vi "Digilens DLP Gen2 UI .vi"(11 "TopLevel In":refnum<class "TopLevel.lvclass">) -> (3 "TopLevel Out":refnum<class "TopLevel.lvclass">)   [LabVIEW 2022 SP3, in "TopLevel.lvclass"] (continued)
  T26 = typedef "TopLevel.lvclass/API Command Enum.ctl" = enum16{"Execute Printer Commands", "Pre Purge", "Enable Ink Ch-1", "Enable Ink Ch-2", "Enable Ink Ch-3", "Enable Ink Ch-4", "Enable Ink Ch-5", "Enable Ink Ch-6", "Disable Ink Ch-1", "Disable Ink Ch-2", "Disable Ink Ch-3", "Disable Ink Ch-4", "Disable Ink Ch-5", "Disable Ink Ch-6", "ExecuteIdlePrintCycle", "StopIdlePrintCycle", "Abort", "LoadDLP2GUIConfig", "SaveDLP2GUIConfig", "PrimingMode", "SetHeadTemperature", "EnableHead", "EnableHeadHeat", "SetSystemMode", "HeadPrint", "AbortAll", "Send Printer String", "WriteInitXML"}
  T27 = typedef "TopLevel.lvclass/PrimingMode APIData.ctl" = cluster{"Interval (s)":dbl, "PurgeDuration (s)":dbl, "Repeats":u8, "PrimingMode":T13, "Head":T18, "Frequency (Hz)":i32, "PrintWeight":dbl}
  T28 = typedef "PrintCmdParameters--Cluster.ctl" = cluster{"Command File Path":path, "No. of Print Repeats":i32, "HomeOnComplete":bool}
  T29 = typedef "TopLevel.lvclass/API Command Cluster.ctl" = cluster{"Command":T26, "Arguments":string, "Data":variant}
  T30 = typedef "IdlePrintCmdParameters--Cluster.ctl" = cluster{"Command File Path":path, "IdleMode":bool, "IdleCycleInterval(s)":dbl}
  T31 = typedef "IO.lvclass/ICP2-DO Channel Names.ctl" = enum16{"None", "Meniscus Valve Open - R1", "Meniscus Valve Open - R2", "Meniscus Valve Open - R3", "Meniscus Valve Open - R4", "Meniscus Valve Open - R5", "Meniscus Valve Open - R6", "Ink Flow Valve Open - R1", "Ink Flow Valve Open - R2", "Ink Flow Valve Open - R3", "Ink Flow Valve Open - R4", "Ink Flow Valve Open - R5", "Ink Flow Valve Open - R6", "SW_LED - Ink Valve - R1", "SW_LED - Ink Valve - R2", "SW_LED - Ink Valve - R3", "Recirc Pump On - R1", "Recirc Pump On - R2", "Recirc Pump On - R3", "Recirc Pump On - R4", "Recirc Pump On - R5", "Recirc Pump On - R6", "SW_LED - Ink Valve - R4", "SW_LED - Ink Valve - R5", "SW_LED - Ink Valve - R6"}
  T32 = enum32{"invalid app kind", "Development System", "Run Time System", "Student Edition", "Embedded LabVIEW", "Evaluation", "Custom"}
  T33 = typedef "printWeights--cluster.ctl" = cluster{"Weights 1":dbl, "Weights 2":dbl, "Weights 3":dbl, "Weights 4":dbl, "Weights 5":dbl, "Weights 6":dbl}
  T34 = typedef "Imageresolution--cluster.ctl" = cluster{"X Resolution":i32, "Y Resolution":i32}
  T35 = typedef "TD MasterConfiguration DLPC2--cluster.ctl" = cluster{"Paths":T36, "ColorPaneMapping":T37, "Materials":string[], "ColorPlanes":string[], "SpitVoltages_Half":T39, "SpitVoltages_Full":T39, "SystemMode":string[], "PrimeModeConfig":T27[], "Running Average Duration_s":dbl}
  T36 = typedef "DLPC2_Path--Cluster.ctl" = cluster{"DigiBit WG Design Folder":path, "Compensated GS Image Folder":path, "Nozzle GS Files Head 1":path, "Nozzle GS Files Head 2":path, "Nozzle GS Files Head 3":path, "Nozzle GS Files Head 4":path, "Nozzle GS Files Head 5":path, "Nozzle GS Files Head 6":path}
  T37 = typedef "TD HeadColorPaneMappingAll--cluster.ctl" = cluster{"Head 1":T38, "Head 2":T38, "Head 3":T38, "Head 4":T38, "Head 5":T38, "Head 6":T38}
  T38 = typedef "TD HeadColorPaneMapping--cluster.ctl" = cluster{"Material":string, "ColorPane":string}
  T39 = typedef "SpitVoltages--Cluster.ctl" = cluster{"1":dbl, "2":dbl, "3":dbl, "4":dbl, "5":dbl, "6":dbl}
  T40 = typedef "Motor Controller.lvclass/Status.ctl" = cluster{"Motor Controller Config Data":T41, "Motor Controller Data":cluster{"Enabled?":bool}, "Stage Move":T42, "Stage Busy?":bool}
  T41 = typedef "Motor Controller.lvclass/Motor Controller Config Data.ctl" = cluster{"Motor IP Addresss":string, "Current Position":i32, "Pulse_Per_mm":i32, "PrePrint":dbl[], "Load Position_mm":i32, "Laminate Position_mm":i32}
  T42 = typedef "Motor Controller.lvclass/Stage Move Data.ctl" = cluster{"Current Step":string, "Move Data":T43[]}
  T43 = typedef "Motor Controller.lvclass/Batch Index Speed Data.ctl" = cluster{"Batch & Cycle":string, "Move":cluster{"Index_mm":i32, "Speed_mm_s":i32}, "Status":T44}
  T44 = typedef "Motor Controller.lvclass/Move Status.ctl" = enum16{"Pending", "In Progress", "Completed"}
  T45 = enum8{"Enabled", "Disabled", "Disabled and Grayed Out"}
  T46 = enum32{"Invalid", "Standard", "Closed", "Hidden", "Minimized", "Maximized"}
  T47 = typedef "LoadImagesData--cluster.ctl" = cluster{"Images[]":path[], "Calibration":bool}
  T48 = typedef "PythonVersion--Enum.ctl" = enum16{"3.9 64", "3.9 32", "3.12 64", "3.12 32"}
  T49 = typedef "SeperateLayersPython--cluster.ctl" = cluster{"Path_to_Tiff":path, "OutputFolder":path, "DPI_x":i32, "DPI_y":i32, "Python_Version":T48}
  T50 = typedef "IO.lvclass/ICP1-AO Channel Names.ctl" = enum16{"None", "Meniscus Pressure Set - R1", "Meniscus Pressure Set - R2", "Meniscus Pressure Set - R3", "Meniscus Pressure Set - R4", "Meniscus Pressure Set - R5", "Meniscus Pressure Set - R6", "Meniscus Vac Pump Speed"}
  T51 = typedef "TopLevel.lvclass/Digilens Config Cluster.ctl" = cluster{"Motion Controller":T41, "IO Config":T52, "PrinterConfiguration":T55, "DAQ Settings":T56}
  T52 = typedef "IO.lvclass/IO Config Data.ctl" = cluster{"DAQDevices":T53[], "DI Channels":T54[], "DO Channels":T54[], "Material Names":string[], "AI Channels":T54[], "AO Channels":T54[]}
  T53 = typedef "IO.lvclass/DCON_DeviceConfig--Cluster.ctl" = cluster{"COM":string, "DeviceName":string, "BaudRate":u32, "Number of Channels":i32, "DeviceAddress":i32, "Enable":bool}
  T54 = typedef "IO.lvclass/Channel Data.ctl" = cluster{"Channel Name":string, "Device Name":string, "Channel No":string}
  T55 = typedef "GIS Printer.lvclass/PrinterConfiguration--Cluster.ctl" = cluster{"IPAddress":string, "Move Stage on RTP Command?":bool, "Stage Move Position":string, "PH1-Prime Path":path, "PH2-Prime Path":path, "PH3-Prime Path":path, "PH4-Prime Path":path, "PH5-Prime Path":path, "PH6-Prime Path":path, "PrintScriptsFolder":path, "PurgeScriptsFolder":path, "StageScriptsFolder":path, "PH1-HeatOn Path":path, "PH2-HeatOn Path":path, "PH3-HeatOn Path":path, "PH4-HeatOn Path":path, "PH5-HeatOn Path":path, "PH6-HeatOn Path":path, "PH1-HeatOff Path":path, "PH2-HeatOff Path":path, "PH3-HeatOff Path":path, "PH4-HeatOff Path":path, "PH5-HeatOff Path":path, "PH6-HeatOff Path":path}
  T56 = typedef "DAQ.lvclass/TD DAQ Settings--cluster.ctl" = cluster{"Simulate DAQ":bool, "DI Settings":T57[], "AI Settings":T58[], "Relay IONames":string[], "AO IONames":string[], "AO NChan SingleTask":bool}
  T57 = typedef "DAQ.lvclass/TD DI Instrument Settings--cluster.ctl" = cluster{"Disable":bool, "DI TaskName":string, "DI RefreshIntv":i32}
  T58 = typedef "DAQ.lvclass/TD AI Instrument Settings--cluster.ctl" = cluster{"Disable":bool, "AI TaskName":string, "AI InstSettings":T59, "SimAI Ranges":T60}
  T59 = typedef "DAQ.lvclass/TD AI InstSettings--cluster.ctl" = cluster{"DaqRate":dbl, "NumSamples":i32}
  T60 = typedef "DAQ.lvclass/TD SimAI Ranges--cluster.ctl" = cluster{"lo":dbl, "hi":dbl}
  T61 = typedef "DLPConfig_Initialization.ctl" = cluster{"PrinterInitialization":cluster{"Printer":cluster{"#attributes":cluster{"Name":string}}, "VacPumpSet":cluster{"#attributes":cluster{"VacPumpEnable":bool, "VacPumpSpeed":dbl}}, "HIBEnable":cluster{"#attributes":cluster{"HIB1Enable":bool, "HIB2Enable":bool, "HIB3Enable":bool, "HIB4Enable":bool, "HIB5Enable":bool, "HIB6Enable":bool}}, "PrinterCompensation":T62}, "HeadSet":cluster{"HeadProperties":T63[]}, "InkSet":cluster{"Ink":T65[]}, "Troubleshooting":cluster{"PMBLogging":cluster{"#attributes":cluster{"PMBMonitorDuringPrint":bool, "PMBMonitorDuringIdle":bool, "LogSwatheInputData":bool, "LogSwatheOutputData":bool, "LogPrintheadColourPlanes":bool, "LogPMBCommunication":bool, "LogSimulatedOutput":bool, "LogAllPMBCommunicationData":bool, "LogPMBSpace":bool, "ExtendedPMBSpaceLogging":bool, "LogPMBWriteSpeed":bool, "LogUsbRetries":bool}}, "HIBLogging":cluster{"#attributes":cluster{"HIBMonitoringDuringPrint":bool, "HIBMonitoringLog":bool}}}}
  T62 = typedef "DLP2_PrinterCompensationProperties.ctl" = cluster{"#attributes":cluster{"AppName":string, "PrintWeightMultiplier":dbl, "Rotation":bool, "Driver":string, "Server":string, "Database":string, "User":string, "Password":string}}
  T63 = typedef "DLP2_PrinterHeadProperties.ctl" = cluster{"#attributes":T64}
  T64 = typedef "DLPConfig)Init_HeadPropertyAttr--Cluster.ctl" = cluster{"HeadNumber":u8, "Material":string, "HeadLocalX":dbl, "HeadLocalY":dbl, "HeadRotationAngle":dbl, "VH2L_Hi":dbl, "VH2R_Hi":dbl, "VH1LA_Hi":dbl, "VH1LB_Hi":dbl, "VH1RA_Hi":dbl, "VH1RB_Hi":dbl, "VH2L_Lo":dbl, "VH2R_Lo":dbl, "VH1LA_Lo":dbl, "VH1LB_Lo":dbl, "VH1RA_Lo":dbl, "VH1RB_Lo":dbl}
  T65 = typedef "DLP2_PrinterMaterialProperties.ctl" = cluster{"#attributes":cluster{"InkType":string, "ColorPlane":string, "Heat":dbl, "Meniscus":dbl, "Recirculation":bool, "PrePrintPurge":bool, "PurgeTime":dbl, "PurgeCount":i32, "Density":dbl, "NumberofDrops":i32, "PrintWeight":dbl, "PrintheadPrime":bool}, "Idle":T66}
  T66 = typedef "InkIdleNodeConfigXML--Cluster.ctl" = cluster{"ShortIdle":cluster{"#attributes":cluster{"Heat":dbl, "Meniscus":dbl, "Recirculation":bool}}, "LongIdle":cluster{"#attributes":cluster{"Heat":dbl, "Meniscus":dbl, "Recirculation":bool}}}
  T67 = typedef "TopLevel.lvclass/Pre Purge Parameters.ctl" = cluster{"GIS File Path":path, "Duration (s)":dbl, "No. of Repeats":i32}
  T68 = typedef "RecipeInfo--Cluster.ctl" = cluster{"Path":path, "Type":string, "Product":string}
  T69 = typedef "TiffImageData--Cluster.ctl" = cluster{"ImageBufferMain":u8[][], "ChannelTargetMaterials":string[], "MaterialNames":string[]}
  T70 = typedef "GIS Status--Cluster.ctl" = cluster{"HeadEnabled":bool, "SpitEnabled":bool, "HeaterEnabled":bool, "TargetTemperature":dbl, "CurrentTemperature":dbl}
  T71 = typedef "HeadEnableStatus--cluster.ctl" = cluster{"PH1_Enable":bool, "PH2_Enable":bool, "PH3_Enable":bool, "PH4_Enable":bool, "PH5_Enable":bool, "PH6_Enable":bool}
  T72 = typedef "PersistentData--Cluster.ctl" = cluster{"ToolIdle":bool, "Meniscus Vac Pump Speed":dbl, "InkChEnable":cluster{"Enable Ink Ch-1":bool, "Enable Ink Ch-2":bool, "Enable Ink Ch-3":bool, "Enable Ink Ch-4":bool, "Enable Ink Ch-5":bool, "Enable Ink Ch-6":bool}, "HeatEnable":cluster{"Heater-1 Off":bool, "Heater-2 Off":bool, "Heater-3 Off":bool, "Heater-4 Off":bool, "Heater-5 Off":bool, "Heater-6 Off":bool}, "MiniscusPressure":cluster{"Meniscus Pressure Set - R1":dbl, "Meniscus Pressure Set - R2":dbl, "Meniscus Pressure Set - R3":dbl, "Meniscus Pressure Set - R4":dbl, "Meniscus Pressure Set - R5":dbl, "Meniscus Pressure Set - R6":dbl}, "RecircPumpFlow":cluster{"Recirc Pump Flow Set - R1":dbl, "Recirc Pump Flow Set - R2":dbl, "Recirc Pump Flow Set - R3":dbl, "Recirc Pump Flow Set - R4":dbl, "Recirc Pump Flow Set - R5":dbl, "Recirc Pump Flow Set - R6":dbl}}
  T73 = typedef "DLPConfig_RecipePrints.ctl" = cluster{"CellPrintRecipe":cluster{"#attributes":cluster{"Type":string, "RecipeName":string, "Product":string}, "CellPrint":cluster{"#attributes":cluster{"PrintImageFile":string, "PrintPass":i32, "PrintMode":string, "EncoderSource":string, "PrintGoSource":string, "DitheredSavePath":string, "GSSavePath":string}}[], "InkCompensationSet":cluster{"InkCompensation":cluster{"#attributes":cluster{"InkType":string, "Waveform":string, "ZoneCompensation":bool, "ZoneCompFile":string, "Overprint":dbl, "Bitmap":string, "SaveGSImg":bool, "GSSource":string, "GSValFile":string}}[]}}}
  T74 = typedef "DLPConfig_CalibrationPrints.ctl" = cluster{"CellPrintRecipe":cluster{"#attributes":cluster{"Type":string, "RecipeName":string, "Product":string}, "CellPrint":cluster{"#attributes":cluster{"PrintImageFile":string, "PrintPass":i32, "EncoderSource":string, "PrintGoSource":string, "Head":i32}}[], "InkCompensationSet":cluster{"InkCompensation":cluster{"#attributes":cluster{"InkType":string, "Waveform":string, "ZoneCompensation":bool}}[]}}}
  T75 = typedef "LoginEventData--CLuster.ctl" = cluster{"UserLevel":T76, "Login Time":timestamp}
  T76 = typedef "UserLevel--Enum.ctl" = enum16{"None", "Operator", "Engineer"}
  T77 = cluster{"Core":cluster{"Current VI Reference":refnum<vi>, "Close Panel on Exit?":bool}, "IO":refnum<class "IO.lvclass">, "GIS Printer":refnum<class "GIS Printer.lvclass">, "Motor Controller":refnum<class "Motor Controller.lvclass">, "Methods:Accessors:Digilens Config":T51, "Methods:Accessors:PrinterInitializationXML":T61, "Status":T40, "Exit Event":refnum<user-event>, "Purge\\PrePurge Channel Name":T19, "Pre Purge Parameters":T67, "API Command":T26, "TopLevel out":refnum<class "TopLevel.lvclass">, "Database":refnum<class "Database.lvclass">, "DLP2":refnum<class "DLP2.lvclass">, "DLP2Config":T35, "Materials":string[], "Color Panes":string[], "ConfigSaveRequired":bool, "DLP2ConfigLoaded":T35, "PrintDesign":T68, "DAQ":refnum<class "DAQ.lvclass">, "RGB Image":T6, "Planes Image":T6, "TIFFImageData":T69, "Image Resolution":T34, "Pre Purge API Data":T27, "Prime Names":cluster{"Prime 1":string, "Prime 2":string, "Prime 3":string, "Prime 4":string, "Prime 5":string, "Prime 6":string}, "Heater Enable":cluster{"HeaterEnblHead":T18, "Enable":bool}, "Head Temp ":cluster{"Head 1":cluster{"Actual":dbl, "Target":dbl}, "Head 2":cluster{"Actual":dbl, "Target":dbl}, "Head 3":cluster{"Actual":dbl, "Target":dbl}, "Head 4":cluster{"Actual":dbl, "Target":dbl}, "Head 5":cluster{"Actual":dbl, "Target":dbl}, "Head 6":cluster{"Actual":dbl, "Target":dbl}}, "GISHeadStatus":T70[], "SettingsUpdate":variant, "HeadStatus":T71, "Methods:Accessors:ConfigDict":T16, "Print":cluster{"RecipeXMLPath":path}, "SeparateLayers":T49, "PersistentData":T72, "HeadStatusPollData":T71, "CurrentDLPRecipe":T73, "CalibrationPrints":T74, "Login":T75, "PrintWeights":T33, "PrePrimeDone":bool, "PrePrimeTmrEnabled":bool, "PPP_Ditherered_Images":path[]}
  T78 = enum16{"Left Button", "Center Button", "Right Button", "Window Close"}
  T79 = typedef "eventvkey.ctl" = enum16{"ASCII", "Enter", "Return", "Shift", "Ctrl", "Alt", "Cmd", "Opt", "Caps", "NumLock", "Clear", "Break", "Up", "Down", "Left", "Right", "Insert", "Delete", "Home", "End", "PageUp", "PageDown", "Escape", "Help", "Pause", "ScrollLock", "F1", "F2", "F3", "F4", "F5", "F6", "F7", "F8", "F9", "F10", "F11", "F12", "F13", "F14", "F15", "F16", "F17", "F18", "F19", "F20", "F21", "F22", "F23", "F24", "Play", "VolumeUp", "VolumeDown", "Mute", "Two Byte Char"}
  T80 = typedef "NI_LVConfig.lvlib/Config Data RefNum.ctl" = refnum<k1>
  T81 = cluster{"#attributes":cluster{"PrintImageFile":string, "PrintPass":i32, "EncoderSource":string, "PrintGoSource":string, "Head":i32}}[]
  T82 = cluster{"PrintImageFile":string, "PrintPass":i32, "EncoderSource":string, "PrintGoSource":string, "Head":i32}
  T83 = typedef "TD Pathnames--cluster.ctl" = cluster{"RunTimeSys?":bool, "AppFolder":path, "ExecutablePath":path, "ConfigFolder":path, "DataLogFolder":path, "SystemLogFolder":path, "SeqFolder":path, "MainStartupPathname":path, "MainUIPathname":path, "SystemEventsFile":path, "SeqEventsFile":path, "Config SettingsFile":path, "DAQ IOConfigFile":path, "SystemSimulation":bool, "DLPUIConfigFile":path, "PrinterInitXMLFile":path, "PersistentXMLFile":path, "Error Log Folder":path, "RecipeXMLFolder":path, "CalibrationRecipeXMLFolder":path}
  T84 = typedef "DLP RecipeTypesData--Cluster.ctl" = cluster{"Product":string, "RecipePathsByProduct":path[], "RecipeNamesByProduct":string[]}
  T85 = typedef "DLP_MaterialToHeadMapping--Cluster.ctl" = cluster{"Head":u8, "Ink":T65}
  T86 = cluster{"Head 1":cluster{"Actual":dbl, "Target":dbl}, "Head 2":cluster{"Actual":dbl, "Target":dbl}, "Head 3":cluster{"Actual":dbl, "Target":dbl}, "Head 4":cluster{"Actual":dbl, "Target":dbl}, "Head 5":cluster{"Actual":dbl, "Target":dbl}, "Head 6":cluster{"Actual":dbl, "Target":dbl}}
  T87 = cluster{"Current VI Reference":refnum<vi>, "Close Panel on Exit?":bool}
  T88 = typedef "TopLevel.lvclass/UserEvents.ctl" = cluster{"API Incoming Event":refnum<user-event>, "API Executed Event":refnum<user-event>, "API Return Event":refnum<user-event>, "Exit Event":refnum<user-event>, "StatusChanged":refnum<user-event>, "DLP GUI Config Changed":refnum<user-event>, "AppEvent":refnum<user-event>, "Login Event":refnum<user-event>, "HeadPrimeStatusEvent":refnum<user-event>}
  T89 = cluster{"Prime 1":string, "Prime 2":string, "Prime 3":string, "Prime 4":string, "Prime 5":string, "Prime 6":string}
  T90 = typedef "Image Type" = u32
  T91 = enum8{"Enabled", "Disabled", "Disabled and Grayed Out"}[]
  T92 = cluster{"#attributes":cluster{"PrintImageFile":string, "PrintPass":i32, "PrintMode":string, "EncoderSource":string, "PrintGoSource":string, "DitheredSavePath":string, "GSSavePath":string}}[]
  T93 = cluster{"#attributes":cluster{"PrintImageFile":string, "PrintPass":i32, "PrintMode":string, "EncoderSource":string, "PrintGoSource":string, "DitheredSavePath":string, "GSSavePath":string}}
  T94 = typedef "DLP2.lvclass/Public Events--cluster.ctl" = cluster{"Temp01.AsyncCmd Event":refnum<user-event>, "Temp01.AsyncMsg Event":refnum<user-event>, "stop process":refnum<user-event>, "API Incoming Event":refnum<user-event>, "API Executed Event":refnum<user-event>, "API Return Event":refnum<user-event>, "Images":refnum<user-event>}
  T95 = typedef "Motor Controller.lvclass/UserEvents.ctl" = cluster{"API Incoming Event":refnum<user-event>, "API Executed Event":refnum<user-event>, "API Return Event":refnum<user-event>, "Status Changed Event":refnum<user-event>, "StopEvent":refnum<user-event>}
  T96 = typedef "IO.lvclass/UserEvents.ctl" = cluster{"API Incoming Event":refnum<user-event>, "API Executed Event":refnum<user-event>, "API Return Event":refnum<user-event>, "Status Changed Event":refnum<user-event>}
  T97 = typedef "GIS Printer.lvclass/UserEvents.ctl" = cluster{"API Incoming Event":refnum<user-event>, "API Executed Event":refnum<user-event>, "API Return Event":refnum<user-event>, "Status Changed Event":refnum<user-event>, "Abort":refnum<user-event>, "stop process":refnum<user-event>, "GISPollStatus":refnum<user-event>, "GISHeadStatus":refnum<user-event>, "Error Event":refnum<user-event>}
  T98 = cluster{"HIB1Enable":bool, "HIB2Enable":bool, "HIB3Enable":bool, "HIB4Enable":bool, "HIB5Enable":bool, "HIB6Enable":bool}
  T99 = typedef "processMode_parameters--cluster.ctl" = cluster{"Head Array":u8[], "ProcessHeat[]":dbl[], "ShortIdleHeat[]":dbl[], "LongIdleHeat[]":dbl[], "ProcessMeniscus[]":dbl[], "ShortIdleMeniscus[]":dbl[], "LongIdleMeniscus[]":dbl[], "ProcessRecirc[]":bool[], "ShortIdleRecirc[]":bool[], "LongIdleRecirc[]":bool[]}
  T100 = typedef "RecipesFolderSummary--Cluster.ctl" = cluster{"Products":string[], "RecipeTypes":string[]}
  T101 = typedef "TD IOCtrlUpdate.ctl" = cluster{"IOName":string, "vData":variant}
  T102 = typedef "DAQ.lvclass/TD PublicEvents--cluster.ctl" = cluster{"DaqOutputCmd Ev":refnum<user-event>, "stop process":refnum<user-event>, "DAQ.AsyncCmd Event":refnum<user-event>, "DAQStateChanged Event":refnum<user-event>, "DAQ.AsyncMsg Event":refnum<user-event>, "DAQ_DO_StatusEvent":refnum<user-event>, "DIStateChangeEv":refnum<user-event>, "UI StateChanged":refnum<user-event>, "PurgeTimerEvent":refnum<user-event>}
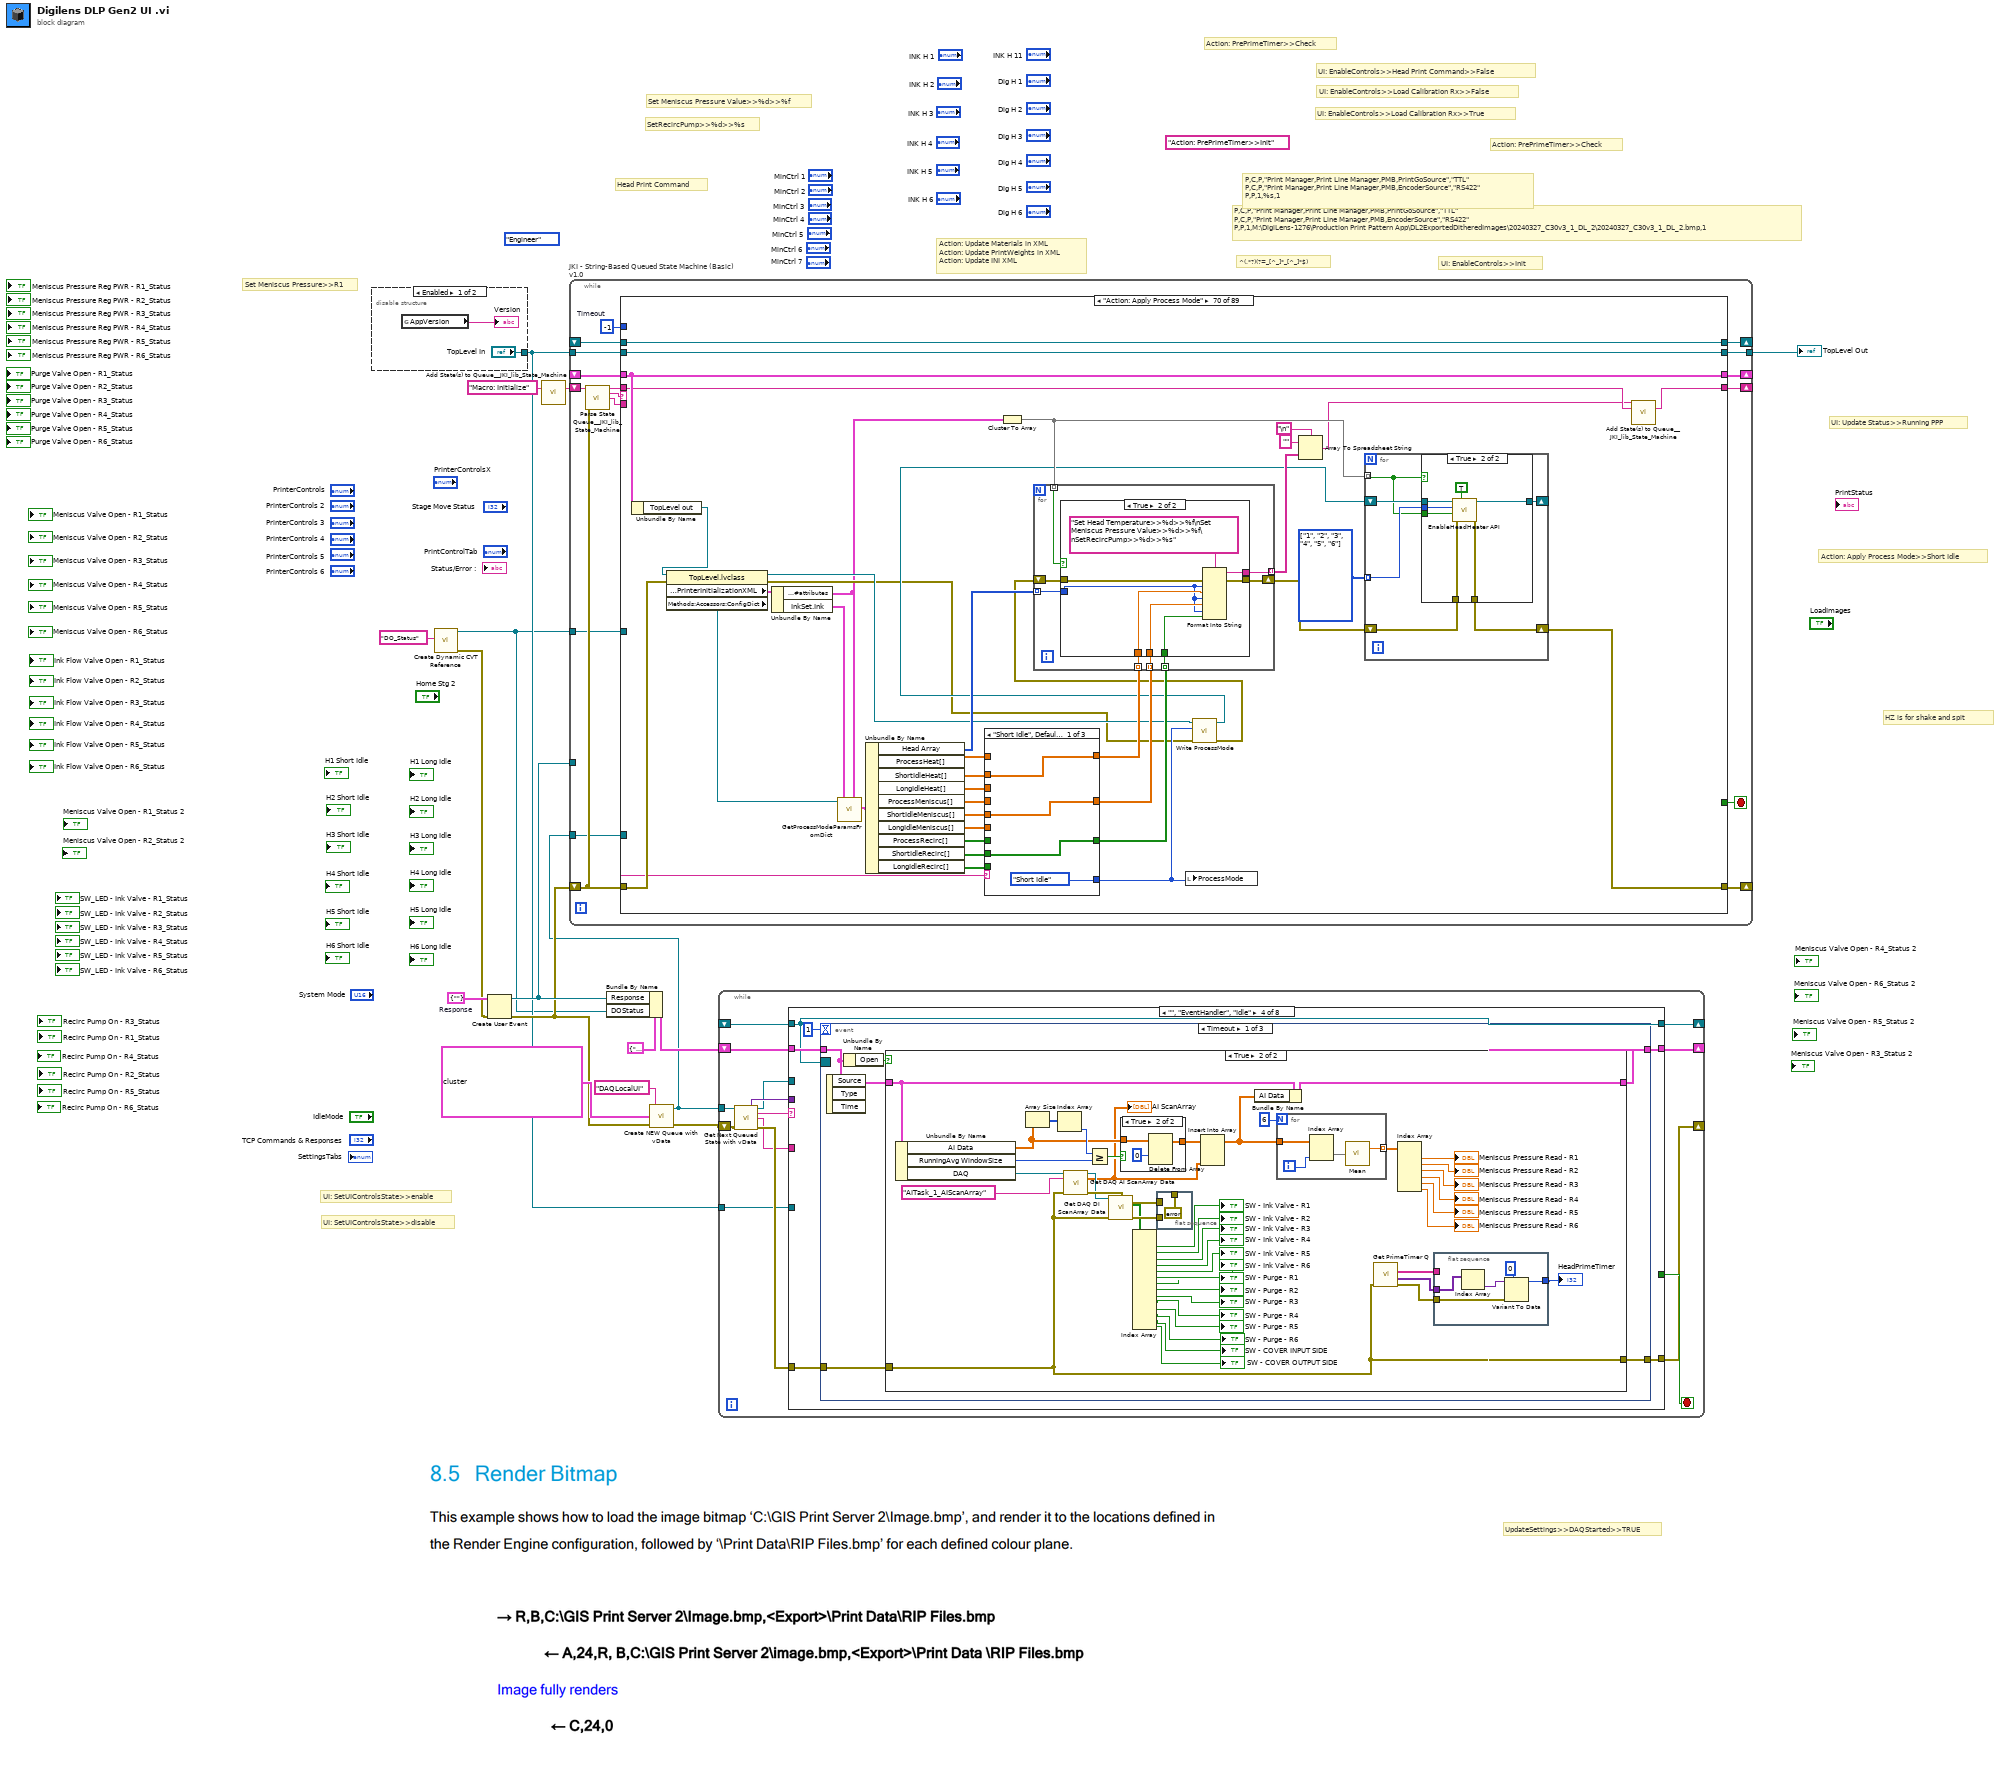
[diagram p0: block diagram]
diagram:
  (unwired) "Action: PrePrimeTimer>>Init" ("State(s) in Front (\"\")")
  (unwired) UserLevel_withoutNone--Enum."Engineer" ("UserLevel")
  w13 = cluster{"Response":string} {"Response"=""}  # Response
  # "SetRecircPump>>%d>>%s"
  # "Set Meniscus Pressure Value>>%d>>%f"
  # "Set Meniscus Pressure>>R1"
  # "Action: Apply Process Mode>>Short Idle"
  # "UI: Update Status>>Running PPP"
  # "UI: EnableControls>>Head Print Command>>False"
  # "Head Print Command"
  # "UI: EnableControls>>Load Calibration Rx>>False"
  # "Action: PrePrimeTimer>>Check"
  # "UI: EnableControls>>Init"
  # "Action: Update Materials in XML\nAction: Update PrintWeights in XML\nAction: Update INI XML"
  # "UI: EnableControls>>Load Calibration Rx>>True"
  # "Action: PrePrimeTimer>>Check"
  # "HZ is for shake and spit"
  # "P,C,P,\"Print Manager,Print Line Manager,PMB,PrintGoSource\",\"TTL\"\nP,C,P,\"Print Manager,Print Line Manager,PMB,EncoderSource\",\"RS422\"\nP,P,1,%s,1"
  # "P,C,P,\"Print Manager,Print Line Manager,PMB,PrintGoSource\",\"TTL\"\nP,C,P,\"Print Manager,Print Line Manager,PMB,EncoderSource\",\"RS422\"\nP,P,1,M:\\DigiLens-1276\\Production Print Pattern App\\DL2ExportedDitheredImages\\20240327_C30v3_1_DL_2\\20240327_C30v3_1_DL_2.bmp,1"
  # "^(.*?)(?=_[^_]*_[^_]*$)"
  # "UpdateSettings>>DAQStarted>>TRUE"
  # "UI: SetUIControlsState>>disable"
  # "UI: SetUIControlsState>>enable"
  n1 = disable-structure shown="Enabled" {
    disable-tunnel: ["TopLevel In" w19] -> w5
    frame Enabled {
      n2 = global read "GBL System.vi" "AppVersion"() -> (→"Version":string)
    }
    frame Disabled {
      n3 = call "Launcher.vi"() -> ("TopLevel out"=w19:refnum<class "TopLevel.lvclass">)  [unwired: 10 in, 1 out]
    }
  }
  n4 = call <vilib>:"Create Dynamic CVT Reference.vi"("DictName"="DO_Status") -> ("error out"=w3:errorcluster, "dCVT DVR out"=w2:T16)  [unwired: 9 in]
  n5 = Create User Event(user event datatype=w13, error in=w3) -> (user event=w7:refnum<user-event>, error out=w6:errorcluster)
  n6 = call <vilib>:"Add State(s) to Queue__JKI_lib_State_Machine.vi"("State(s) in (\"\")"="Macro: Initialize") -> ("States Out"=w16:string)  [unwired: 14 in]
  n7 = Bundle By Name(cluster=T17 {"String"="", "Response"=refnum, "Open"=FALSE, "DAQ"=refnum, "DOStatus"=refnum, "DIStateChangeEv"=refnum, "RunningAvg WindowSize"=0, "AI Data"=[]}, "Response"=w7, "DOStatus"=w2) -> (w8:T17)
  n8 = call <vilib>:"Create NEW Queue with vData.vi"("error in (no error)"=w6, "Initial States"=cluster{"state":string, "vData":variant}[] [{"state"="Initialize", "vData"=variant}, {"state"="Register Events", "vData"=variant}], "Name (SMQ)"="DAQLocalUI") -> ("error out"=w11:errorcluster, "queue out"=w1:refnum<queue>)  [unwired: 1 in]
  n9 = while "JKI - String-Based Queued State Machine (Basic) v1.0" {
    shift-right: [w29] -> _
